vi "DemoArchitecture.vi"() -> ()   [LabVIEW 2018]
uses:
  Global_Sensors.vi
  Global_Commands.vi
panel:
  out "Drive Mode":string
  out "Distance Along Path":dbl
  in  "Sensor 1":bool
  in  "Driver Presses \"B\"":bool
  in  "Driver Presses \"A\"":bool
  in  "Robot Mode":enum16{"Auto", "TeleOp"}(ring)
  out "Subsystem Sequencer":i32
  out "Time Since Latch":u32
  out "J1-B":bool
  out "J1-A":bool
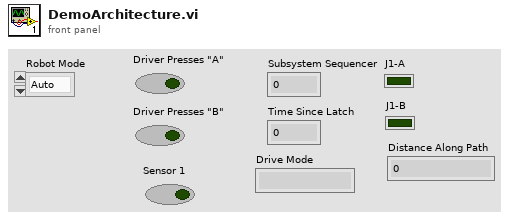
[diagram p1: front panel]
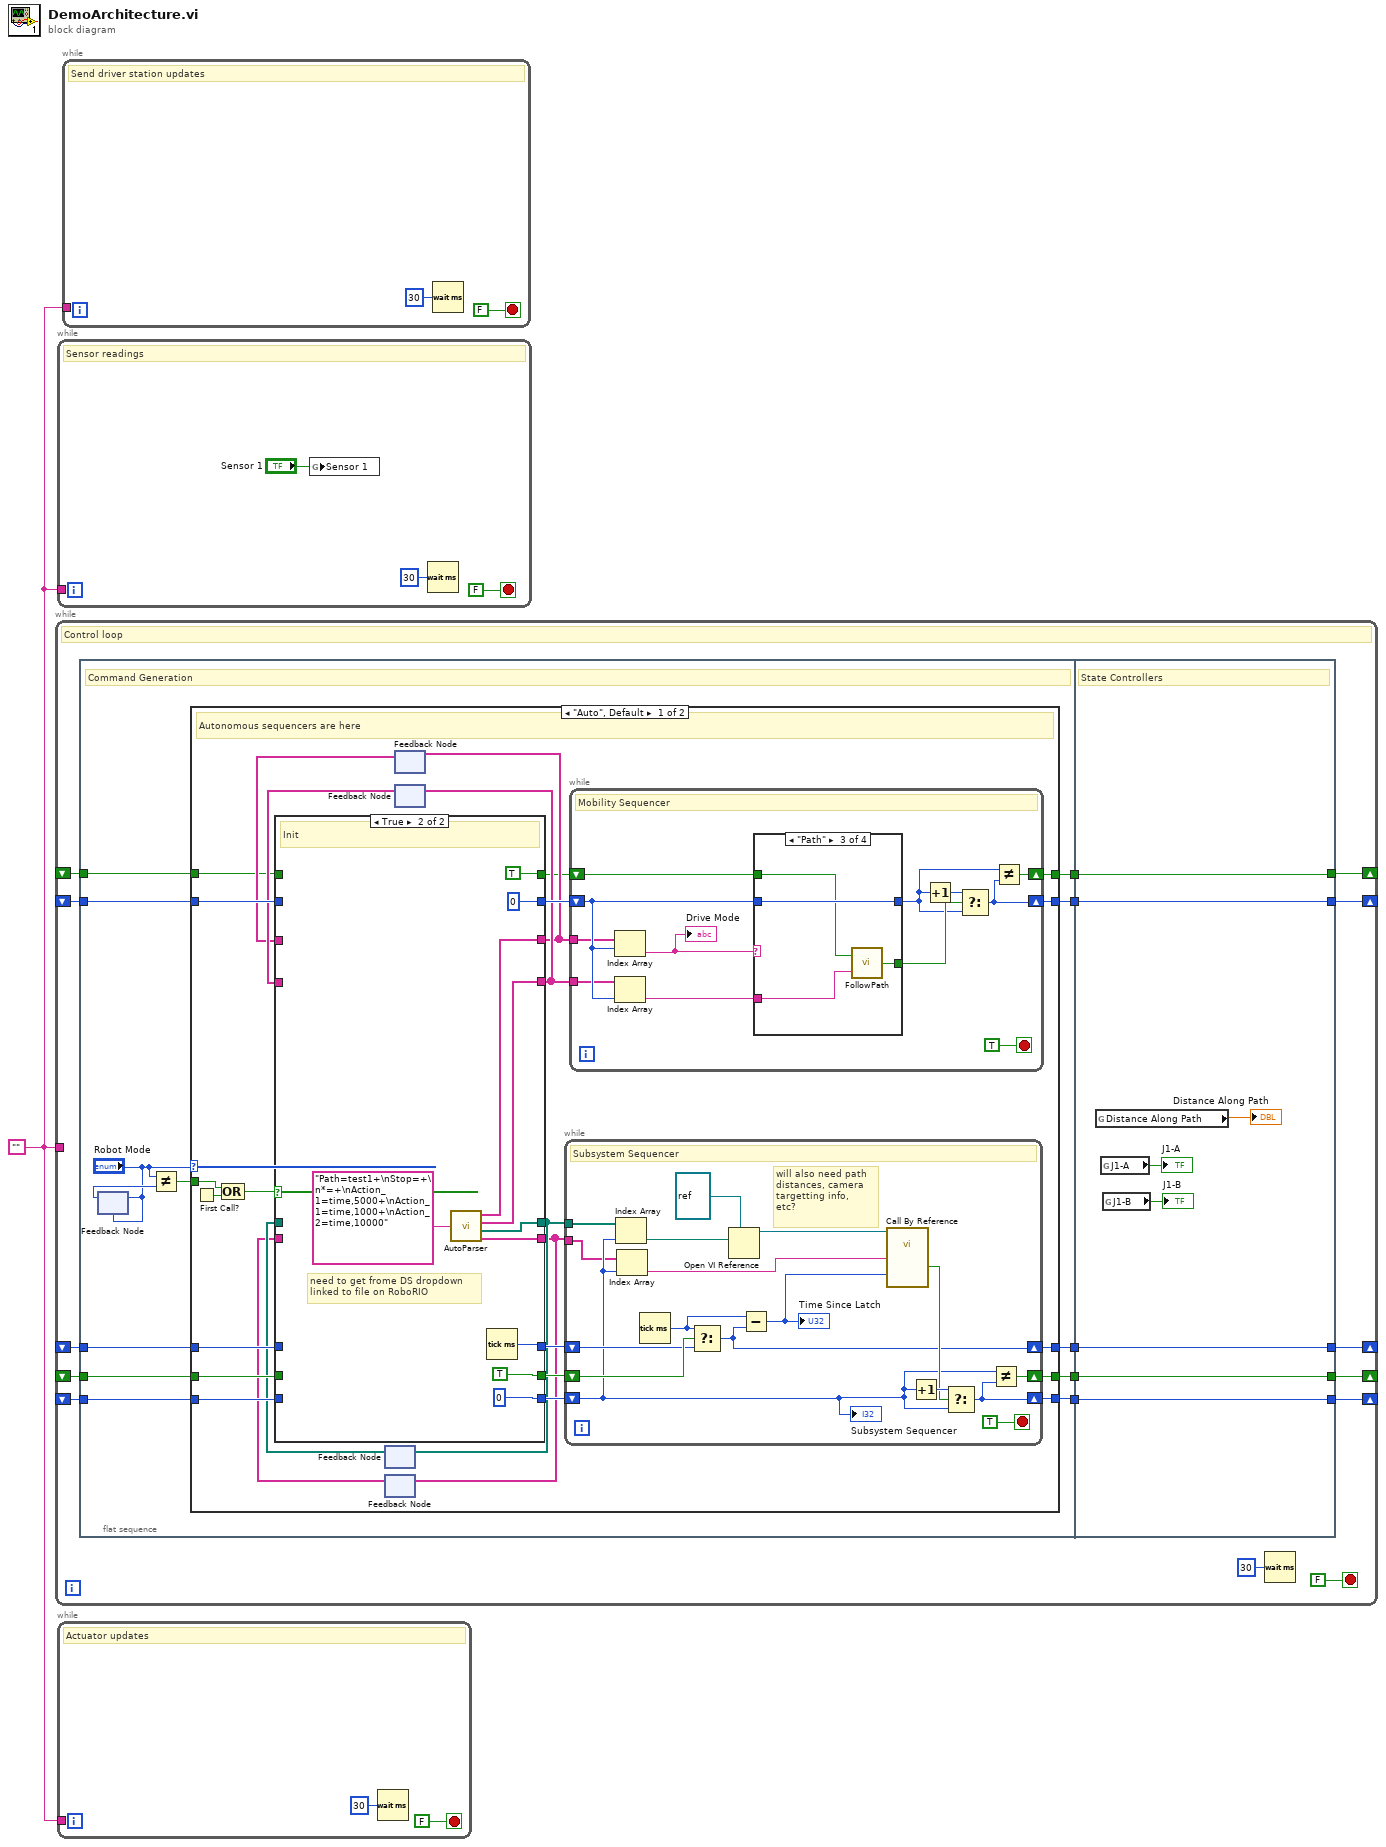
[diagram p0: block diagram]
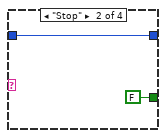
[diagram p3: hidden frame]
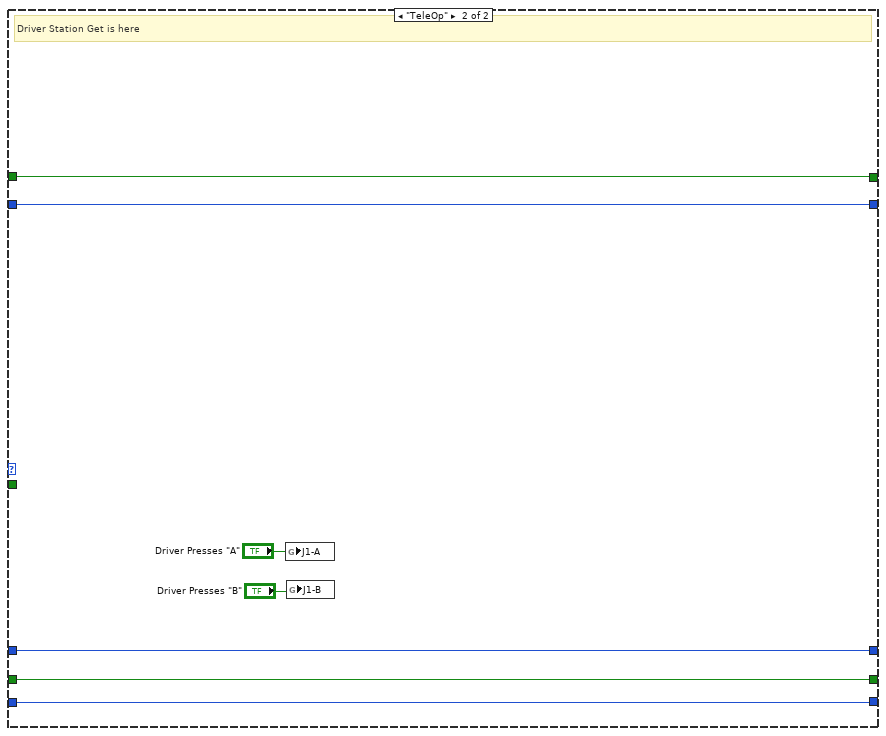
[diagram p6: hidden frame]
diagram:
  w1 = ""
  n1 = while {
    tunnel: w1 -> [_]
    shift-right: [w8] -> _
    shift-left: _ -> [w14]
    shift-right: [w9] -> _
    shift-left: _ -> [w15]
    shift-right: [w10] -> _
    shift-left: _ -> [w16]
    shift-right: [w6] -> _
    shift-left: _ -> [w5]
    shift-right: [w3] -> _
    shift-left: _ -> [w2]
    stop <- FALSE stop-if-true
    # "Control loop"
    n2 = flat-sequence {
      tunnel: w16 -> [w28]
      tunnel: w15 -> [w27]
      tunnel: w14 -> [w26]
      tunnel: [w31] -> w13
      tunnel: [w30] -> w12
      tunnel: [w29] -> w11
      tunnel: [w22] -> w7
      tunnel: w5 -> [w21]
      tunnel: [w20] -> w4
      tunnel: w2 -> [w19]
      tunnel: w13 -> [w126]
      tunnel: w12 -> [w125]
      tunnel: w11 -> [w124]
      tunnel: [w126] -> w10
      tunnel: [w125] -> w9
      tunnel: [w124] -> w8
      tunnel: w7 -> [w122]
      tunnel: [w122] -> w6
      tunnel: [w121] -> w3
      tunnel: w4 -> [w121]
      frame #0 {
        # "Command Generation"
        n3 = feedback-in #1("Robot Mode") -> ()
        n4 = feedback #1("Robot Mode") -> (w25:enum16{"Auto", "TeleOp"})
        n5 = Not Equal?(x="Robot Mode", y=w25) -> (x != y?=w23:bool)
        n6 = case shown="\"Auto\", Default" "Robot Mode" {
          tunnel: w28 -> [w54 w120]
          tunnel: w27 -> [w52 w119]
          tunnel: w26 -> [w51 w118]
          tunnel: [w57 w120] -> w31
          tunnel: [w56 w119] -> w30
          tunnel: [w55 w118] -> w29
          tunnel: w23 -> [w46 _]
          tunnel: [w40 w115] -> w22
          tunnel: w21 -> [w39 w115]
          tunnel: [w33 w114] -> w20
          tunnel: w19 -> [w32 w114]
          frame "Auto", Default {
            # "Autonomous sequencers are here"
            n7 = First Call?() -> (First Call?: T/F=w47:bool)
            n8 = Compound Arithmetic op=OR(w46, w47) -> (w48:bool)
            n9 = feedback #2() -> (w43:path[])  [unwired: 1 in]
            n10 = feedback #3() -> (w42:string[])  [unwired: 1 in]
            n11 = feedback #4() -> (w35:string[])  [unwired: 1 in]
            n12 = feedback #5() -> (w36:string[])  [unwired: 1 in]
            n13 = case shown="True" w48 {
              tunnel: w51 -> [w84 _]
              tunnel: w52 -> [w85 _]
              tunnel: w54 -> [w86 _]
              tunnel: [w86 w96] -> w53
              tunnel: [w85 TRUE ("Advance Trigger")] -> w50
              tunnel: [w84 0] -> w49
              tunnel: [w83 w88] -> w45
              tunnel: [w82 w93] -> w44
              tunnel: w43 -> [w83 _]
              tunnel: w42 -> [w82 _]
              tunnel: [w81 0] -> w41
              tunnel: w39 -> [w81 _]
              tunnel: [w80 w90] -> w38
              tunnel: [w79 w89] -> w37
              tunnel: w36 -> [w80 _]
              tunnel: w35 -> [w79 _]
              tunnel: [w78 TRUE] -> w34
              tunnel: w32 -> [w78 _]
              frame False {
                # "Pass"
              }
              frame True {
                # "need to get frome DS dropdown\nlinked to file on RoboRIO"
                # "Init"
                n14 = call "AutoParser.vi"("Auto Play"="Path=test1+\nStop=+\n*=+\nAction_1=time,5000+\nAction_1=time,1000+\nAction_2=time,10000") -> ("Drive Mode Strings"=w89:string[], "Drive Command Strings"=w90:string[], "Subsystem VI References"=w88:path[], "Subsystem Command Strings"=w93:string[])
                n15 = Tick Count (ms)() -> (millisecond timer value=w96:u32)
              }
            }
            n16 = feedback-in #2(w45) -> ()
            n17 = feedback-in #3(w44) -> ()
            n18 = feedback-in #4(w37) -> ()
            n19 = feedback-in #5(w38) -> ()
            n20 = while {
              tunnel: w45 -> [w101]
              shift-right: [w109] -> w55
              shift-left: w49 -> [w99]
              shift-right: [w108] -> w56
              shift-left: w50 -> [w107]
              shift-right: [w105] -> w57
              shift-left: w53 -> [w106]
              tunnel: w44 -> [w98]
              stop <- TRUE stop-if-true
              # "will also need path \ndistances, camera\ntargetting info, \netc?"
              # "Subsystem Sequencer"
              n21 = Index Array(array=w101, index=w99) -> (element=w100:path)
              n22 = Index Array(array=w98, index=w99) -> (element=w97:string)
              n23 = Tick Count (ms)() -> (millisecond timer value=w104:u32)
              n24 = Select(t=w104, s=w107, f=w106) -> (s? t:f=w105:u32)
              n25 = Open VI Reference(type specifier VI Refnum (for type only)=refnum<vi> refnum, vi path=w100) -> (vi reference=w103:refnum<vi>)  [unwired: 4 in, 1 out]
              n26 = Subtract(x=w104, y=w105) -> (x-y=w102:u32)
              "Time Since Latch" <- w102
              n27 = call-by-ref "?"(reference=w103, "Time Since Latch"=w102, "Instruction String"=w97) -> ("Advance Trigger"=w110:bool)  [unwired: 1 in, 2 out]
              n28 = Increment(x=w99) -> (x+1=w112:i32)
              n29 = Select(t=w112, s=w110, f=w99) -> (s? t:f=w109:i32)
              n30 = Not Equal?(x=w99, y=w109) -> (x != y?=w108:bool)
              "Subsystem Sequencer" <- w99
            }
            n31 = while {
              shift-right: [w61] -> w40
              shift-left: w41 -> [w67]
              tunnel: w37 -> [w66]
              tunnel: w38 -> [w65]
              shift-right: [w60] -> w33
              shift-left: w34 -> [w58]
              stop <- TRUE stop-if-true
              # "Mobility Sequencer"
              n32 = Index Array(array=w66, index=w67) -> (element=w64:string)
              "Drive Mode" <- w64
              n33 = Index Array(array=w65, index=w67) -> (element=w63:string)
              n34 = case shown="\"Path\"" w64 {
                tunnel: w67 -> [w70 w72 w76 w77]
                tunnel: [w70 w72 w76 w77] -> w59
                tunnel: w63 -> [_ _ w74 _]
                tunnel: [_ FALSE ("Increment") w75 _] -> w62
                tunnel: w58 -> [_ _ w73 _]
                frame "Pause", Default {
                }
                frame "Stop" {
                }
                frame "Path" {
                  n35 = call "FollowPath.vi"("Parameter String"=w74, "Reinit"=w73) -> ("Increment"=w75:bool)
                }
                frame "Rotate" {
                }
              }
              n36 = Increment(x=w59) -> (x+1=w68:i32)
              n37 = Select(t=w68, s=w62, f=w59) -> (s? t:f=w61:i32)
              n38 = Not Equal?(x=w59, y=w61) -> (x != y?=w60:bool)
            }
          }
          frame "TeleOp" {
            # "Driver Station Get is here"
            n39 = global write "Global_Commands.vi" "J1-A"("Driver Presses \"A\"") -> ()
            n40 = global write "Global_Commands.vi" "J1-B"("Driver Presses \"B\"") -> ()
          }
        }
      }
      frame #1 {
        # "State Controllers"
        n41 = global read "Global_Sensors.vi" "Distance Along Path"() -> (→"Distance Along Path":dbl)
        n42 = global read "Global_Commands.vi" "J1-A"() -> (→"J1-A":bool)
        n43 = global read "Global_Commands.vi" "J1-B"() -> (→"J1-B":bool)
      }
    }
    n44 = Wait (ms)(milliseconds to wait=u32 30) -> ()  [unwired: 1 out]
  }
  n45 = while {
    tunnel: w1 -> [_]
    stop <- FALSE stop-if-true
    # "Sensor readings"
    n46 = global write "Global_Sensors.vi" "Sensor 1"("Sensor 1") -> ()
    n47 = Wait (ms)(milliseconds to wait=u32 30) -> ()  [unwired: 1 out]
  }
  n48 = while {
    tunnel: w1 -> [_]
    stop <- FALSE stop-if-true
    # "Actuator updates"
    n49 = Wait (ms)(milliseconds to wait=u32 30) -> ()  [unwired: 1 out]
  }
  n50 = while {
    tunnel: w1 -> [_]
    stop <- FALSE stop-if-true
    # "Send driver station updates"
    n51 = Wait (ms)(milliseconds to wait=u32 30) -> ()  [unwired: 1 out]
  }
